vi "Vacuum Switch Panel.vi"() -> ()   [LabVIEW 2021]
uses:
  Classes/Controller/I-O/I-O.lvclass
  Classes/Controller/Controller.lvclass
panel:
  in  "Turn off all":bool
  out "error out":errorcluster
  out "Compression Sensor":bool
  out "Sensor Channel":dbl=6.0
  out "Sensor":bool
  out "sensor pin number":i32=3
  out "tray sensor":bool
  out "secondary valve sensor":bool
  out "primary valve sensor":bool
  in  "Turn on secondary vacuum":bool
  in  "turn on primary vacuum":bool
  in  "secure tray":bool
  out "Valve Channel":dbl=6.0
  in  "Type":enum16{"O ring Vac", "Baseplate Vac"}(ring)
  in  "Position":i32=1 min=1 max=2
  in  "Region":i32=1 min=1 max=2
  in  "On/Off":bool
  in  "Stop":bool
  in  "error in (no error)":errorcluster
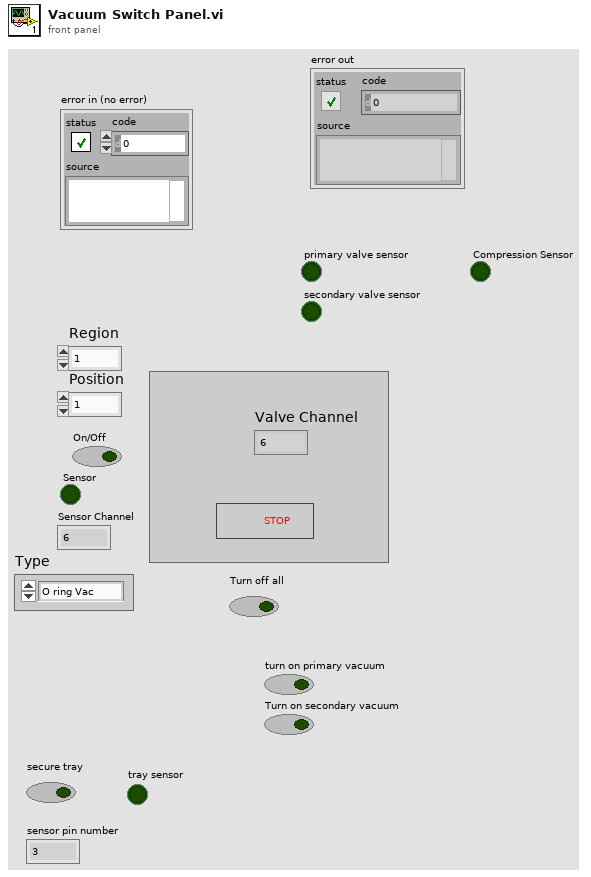
[diagram p1: front panel]
types:
  T1 = typedef "Controller.lvclass/Controllers.ctl" = cluster{"I-O.lvclass":refnum<class "I-O.lvclass">, "Gantry":refnum<k24>, "Dispenser":refnum<visa-resource-name>}
  T2 = typedef "I-O.lvclass/Pin Map.ctl" = cluster{"Region Valves":i32[], "Extra Valves":dbl[][][], "Tool Primary Valve":i32, "Tool Secondary Valve":i32, "Region Sensors":i32[], "Extra Sensors":dbl[][][], "Tool Primary Sensor":dbl, "Tool Secondary Sensor":dbl, "Compression Sensor":dbl, "5V":i32, "Dispenser Sensor":dbl}
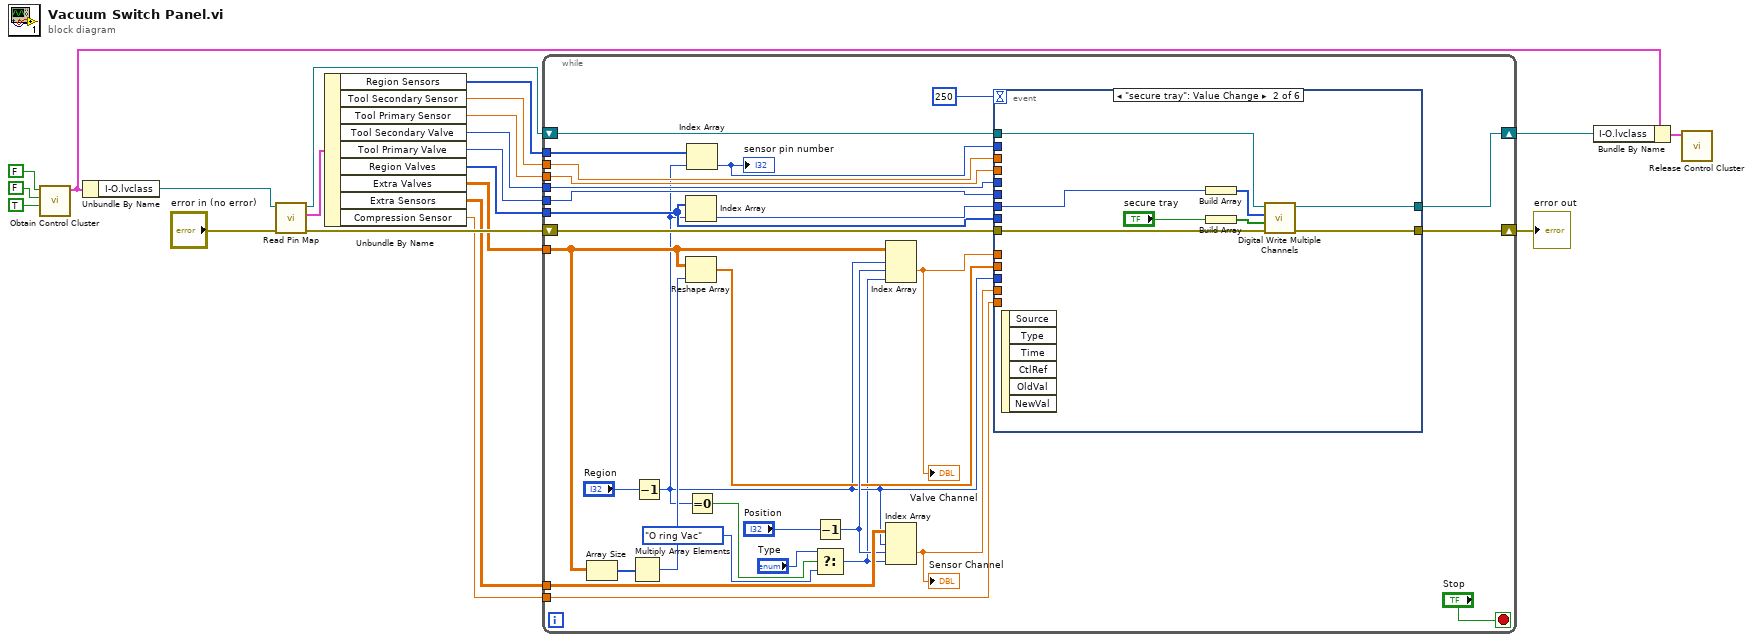
[diagram p0: block diagram]
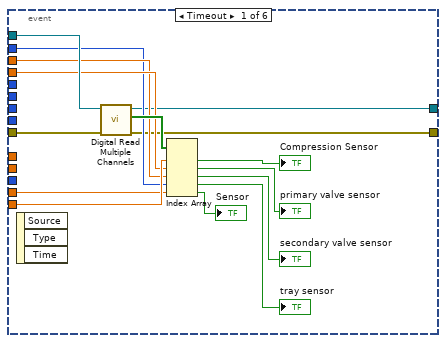
[diagram p2: hidden frame]
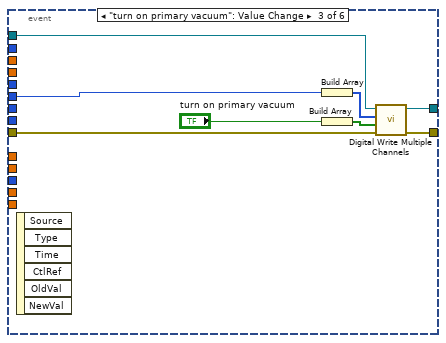
[diagram p3: hidden frame]
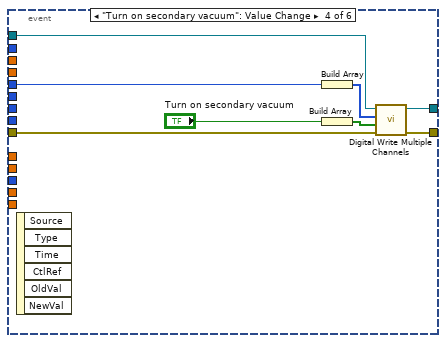
[diagram p4: hidden frame]
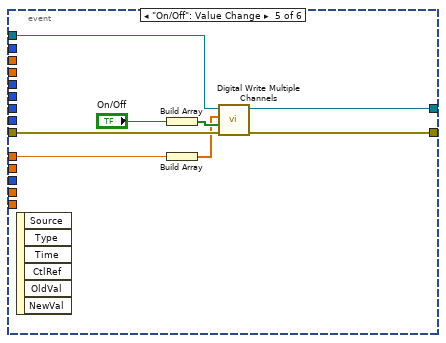
[diagram p5: hidden frame]
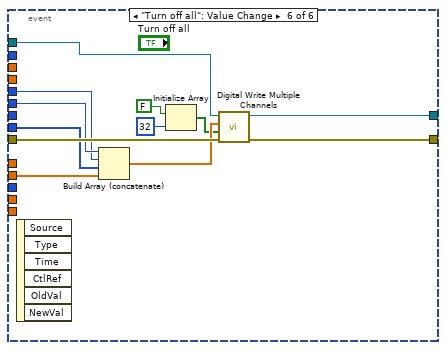
[diagram p6: hidden frame]
diagram:
  n1 = call "Obtain Control Cluster.vi"("I/O"=TRUE, "Dispense"=FALSE, "Motion"=FALSE) -> ("Control Out"=w4:T1)  [unwired: 8 in]
  n2 = Unbundle By Name(w4) -> ("I-O.lvclass"=w17:refnum<class "I-O.lvclass">)
  n3 = call-dynamic "Read Pin Map.vi"("error in (no error)"="error in (no error)", "I-O in"=w17) -> ("error out"=w15:errorcluster, "Pin Map 2"=w21:T2, "I-O out"=w14:refnum<class "I-O.lvclass">)  [unwired: 7 in]
  n4 = Unbundle By Name(w21) -> ("Region Sensors"=w10:i32[], "Tool Secondary Sensor"=w11:dbl, "Tool Primary Sensor"=w12:dbl, "Tool Secondary Valve"=w7:i32, "Tool Primary Valve"=w8:i32, "Region Valves"=w5:i32[], "Extra Valves"=w6:dbl[][][], "Extra Sensors"=w9:dbl[][][], "Compression Sensor"=w13:dbl)
  n5 = while {
    shift-right: [w48] -> w2
    shift-left: w14 -> [w49]
    shift-right: [w47] -> w1
    shift-left: w15 -> [w50]
    tunnel: w10 -> [w44]
    tunnel: w13 -> [w43]
    tunnel: w12 -> [w42]
    tunnel: w11 -> [w41]
    tunnel: w9 -> [w40]
    tunnel: w8 -> [w37]
    tunnel: w7 -> [w36]
    tunnel: w6 -> [w30]
    tunnel: w5 -> [w32]
    stop <- "Stop" stop-if-true
    n6 = Array Size(array=w30) -> (size(s)=w31:i32[])
    n7 = Multiply Array Elements(1:w31) -> (0:w29:i32)
    n8 = Decrement(x="Region") -> (x-1=w26:i32)
    n9 = Index Array(array=w32, index=w26) -> (element=w33:i32)
    n10 = Reshape Array(w30, w29) -> (w28:dbl[])
    n11 = Index Array(array=w44, index=w26) -> (element=w39:i32)
    "sensor pin number" <- w39
    n12 = Equal To 0?(x=w26) -> (x = 0?=w25:bool)
    n13 = Decrement(x="Position") -> (x-1=w35:i32)
    n14 = Select(t="Type", s=w25, f=enum16{"O ring Vac", "Baseplate Vac"}."O ring Vac") -> (s? t:f=w23:enum16{"O ring Vac", "Baseplate Vac"})
    n15 = Index Array(array=w30, index (dim 0)=w26, index (dim 1)=w35, index (dim 2)=w23) -> (element=w34:dbl)
    "Valve Channel" <- w34
    n16 = Index Array(array=w40, index (dim 0)=w26, index (dim 1)=w35, index (dim 2)=w23) -> (element=w38:dbl)
    "Sensor Channel" <- w38
    n17 = event shown="[1] \"secure tray\": Value Change" {
      selector: _ -> [_ _ _ _ _ _]
      dyn-events: _ -> [_ _ _ _ _ _]
      timeout: 250 -> [_ _ _ _ _ _]
      tunnel: w50 -> [w66 w71 w78 w88 w93 w107]
      tunnel: w49 -> [w65 w74 w82 w87 w96 w110]
      tunnel: [w53 w73 w81 w86 w95 w109] -> w48
      tunnel: [w52 w72 w77 w85 w94 w108] -> w47
      tunnel: w26 -> [_ _ _ _ _ _]
      tunnel: w43 -> [w58 _ _ _ _ _]
      tunnel: w42 -> [w57 _ _ _ _ _]
      tunnel: w41 -> [w56 _ _ _ _ _]
      tunnel: w38 -> [w55 _ _ _ _ _]
      tunnel: w39 -> [w54 _ _ _ _ _]
      tunnel: w37 -> [_ _ w76 _ _ w106]
      tunnel: w36 -> [_ _ _ w84 _ w105]
      tunnel: w34 -> [_ _ _ _ w91 _]
      tunnel: w33 -> [_ w68 _ _ _ _]
      tunnel: w32 -> [_ _ _ _ _ w104]
      tunnel: w28 -> [_ _ _ _ _ w103]
      event Timeout {
        n18 = event-data() -> ()  [unwired: 1 in, 3 out]
        n19 = call-dynamic "Digital Read Multiple Channels.vi"("error in (no error)"=w66, "I-O in"=w65) -> ("error out"=w52:errorcluster, "Array 2"=w64:bool[], "I-O out"=w53:refnum<class "I-O.lvclass">)  [unwired: 7 in]
        n20 = Index Array(array=w64, index #1=w58, index #2=w57, index #3=w56, index #4=w54, index #5=w55) -> (element #1=→"Compression Sensor":bool, element #2=→"primary valve sensor":bool, element #3=→"secondary valve sensor":bool, element #4=→"tray sensor":bool, element #5=→"Sensor":bool)
      }
      event "secure tray": Value Change {
        n21 = event-data() -> ()  [unwired: 1 in, 6 out]
        n22 = Build Array(w68) -> (w69:i32[])
        n23 = Build Array("secure tray") -> (w70:bool[])
        n24 = call-dynamic "Digital Write Multiple Channels.vi"("error in (no error)"=w71, "values"=w70, "indices"=w69, "I-O in"=w74) -> ("error out"=w72:errorcluster, "I-O out"=w73:refnum<class "I-O.lvclass">)  [unwired: 6 in]
      }
      event "turn on primary vacuum": Value Change {
        n25 = event-data() -> ()  [unwired: 1 in, 6 out]
        n26 = Build Array(w76) -> (w75:i32[])
        n27 = Build Array("turn on primary vacuum") -> (w79:bool[])
        n28 = call-dynamic "Digital Write Multiple Channels.vi"("error in (no error)"=w78, "values"=w79, "indices"=w75, "I-O in"=w82) -> ("error out"=w77:errorcluster, "I-O out"=w81:refnum<class "I-O.lvclass">)  [unwired: 6 in]
      }
      event "Turn on secondary vacuum": Value Change {
        n29 = event-data() -> ()  [unwired: 1 in, 6 out]
        n30 = Build Array(w84) -> (w83:i32[])
        n31 = Build Array("Turn on secondary vacuum") -> (w90:bool[])
        n32 = call-dynamic "Digital Write Multiple Channels.vi"("error in (no error)"=w88, "values"=w90, "indices"=w83, "I-O in"=w87) -> ("error out"=w85:errorcluster, "I-O out"=w86:refnum<class "I-O.lvclass">)  [unwired: 6 in]
      }
      event "On/Off": Value Change {
        n33 = event-data() -> ()  [unwired: 1 in, 6 out]
        n34 = Build Array("On/Off") -> (w98:bool[])
        n35 = Build Array(w91) -> (w92:dbl[])
        n36 = call-dynamic "Digital Write Multiple Channels.vi"("error in (no error)"=w93, "values"=w98, "indices"=w92, "I-O in"=w96) -> ("error out"=w94:errorcluster, "I-O out"=w95:refnum<class "I-O.lvclass">)  [unwired: 6 in]
      }
      event "Turn off all": Value Change {
        n37 = event-data() -> ()  [unwired: 1 in, 6 out]
        n38 = Build Array (concatenate)(w106, w105, w104, w103) -> (w102:dbl[])
        n39 = Initialize Array(FALSE, 32 ("dimension size")) -> (w99:bool[])
        n40 = call-dynamic "Digital Write Multiple Channels.vi"("error in (no error)"=w107, "values"=w99, "indices"=w102, "I-O in"=w110) -> ("error out"=w108:errorcluster, "I-O out"=w109:refnum<class "I-O.lvclass">)  [unwired: 6 in]
      }
    }
  }
  "error out" <- w1
  n41 = Bundle By Name(cluster=w4, "I-O.lvclass"=w2) -> (w3:T1)
  n42 = call "Release Control Cluster.vi"("output cluster"=w3) -> ()  [unwired: 11 in]
